vi "kalibracja_powerpeak.vi"(6 "mean":dbl, 8 "error in":errorcluster, 9 "Array":dbl[](array[numeric]), 10 "Cursor.Cursor X":dbl, 11 "Cursor.Cursor X 2":dbl) -> (0 "error out":errorcluster, 3 "Est Power peak":dbl=2.5048715520372213e-09 format="%.4e")   [LabVIEW 2013]
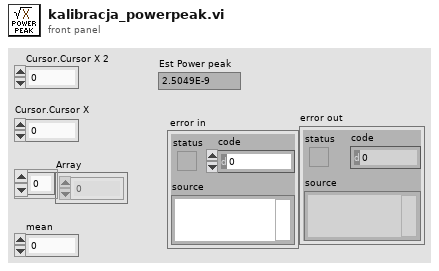
[diagram p1: front panel]
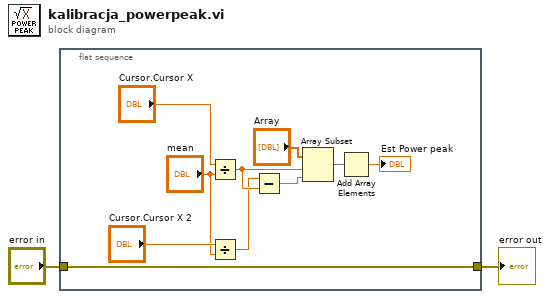
[diagram p0: block diagram]
diagram:
  n1 = flat-sequence {
    tunnel: [w3] -> w1
    tunnel: "error in" -> [w3]
    frame #0 {
      n2 = Divide(x="Cursor.Cursor X", y="mean") -> (x/y=w10:dbl)
      n3 = Divide(x="Cursor.Cursor X 2", y="mean") -> (x/y=w9:dbl)
      n4 = Subtract(x=w9, y=w10) -> (x-y=w11:dbl)
      n5 = Array Subset(array="Array", index=w10, length=w11) -> (w12:dbl[])
      n6 = Add Array Elements(numeric array=w12) -> (sum=→"Est Power peak":dbl)
    }
  }
  "error out" <- w1
